vi "PFI-28000-Overload_Create.vi"(0 "String":string, 11 "error in (no error)":errorcluster) -> (4 "PFI-28000-Overload out":refnum<class "PFI-28000-Overload.lvclass">, 15 "error out":errorcluster)   [LabVIEW 2017, in "PFI-28000-Overload.lvclass"]
uses:
  PFI-28000-Overload.lvclass
  PFI-28000-Overload-Type.ctl
  PFI-28000-Overload.lvclass/PFI-28000-Overload.ctl
  <vilib>/regexp/Match Regular Expression.xnode
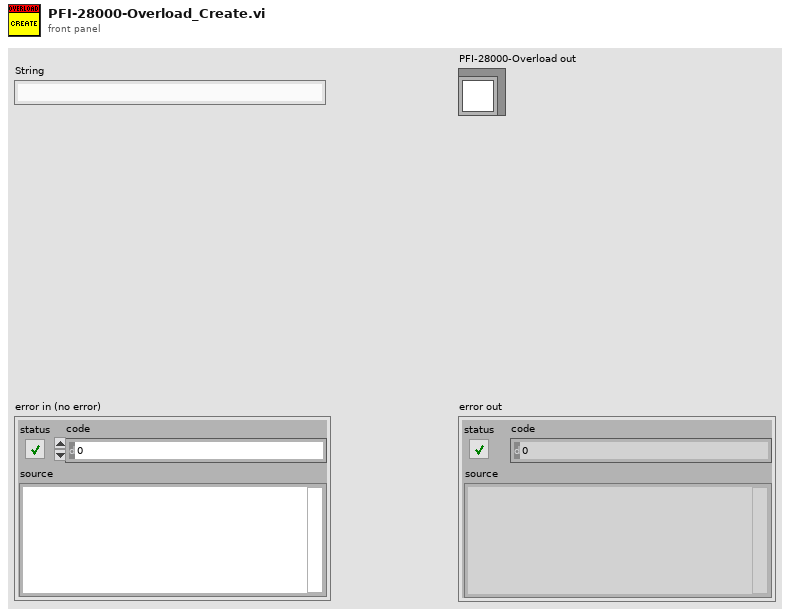
[diagram p1: front panel]
types:
  T1 = typedef "PFI-28000-Overload.lvclass/PFI-28000-Overload-Type.ctl" = enum8{"None", "Filter Input", "Input", "Output", "Open", "Short", "Alarm"}
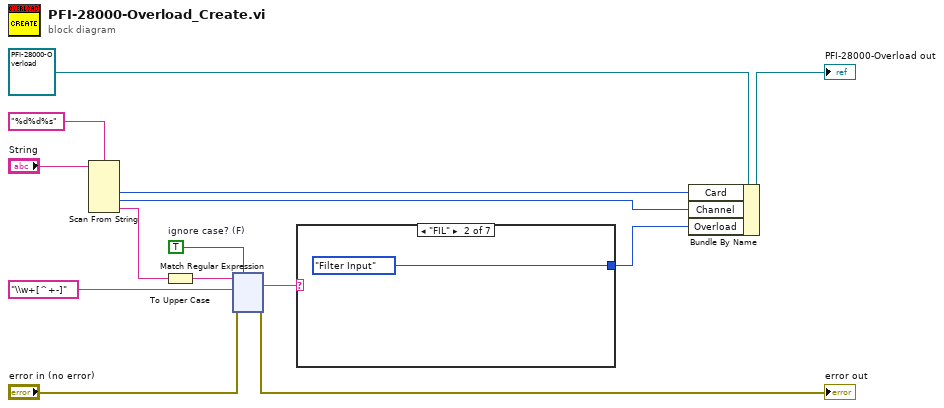
[diagram p0: block diagram]
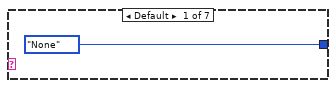
[diagram p2: hidden frame]
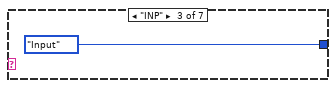
[diagram p3: hidden frame]
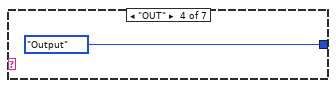
[diagram p4: hidden frame]
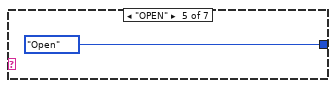
[diagram p5: hidden frame]
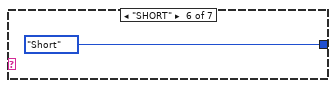
[diagram p6: hidden frame]
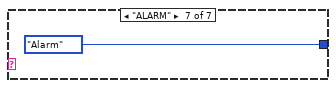
[diagram p7: hidden frame]
diagram:
  w1 = TRUE  # ignore case? (F)
  n1 = Scan From String(format string="%d%d%s" ("empty string"), input string="String") -> (output 1=w11:i32, output 2=w10:i32, output 3=w6:string)  [unwired: 5 in, 3 out]
  n2 = To Upper Case(1:w6) -> (0:w2:string)
  n3 = xnode "Match Regular Expression"("input string"=w2, "regular expression"="\\w+[^+-]" ("empty string"), "error in"="error in (no error)", "ignore case? (F)"=w1) -> ("whole match"=w5:string, "error out"=→"error out":errorcluster)  [unwired: 2 in, 3 out]
  n4 = case shown="\"FIL\"" w5 {
    tunnel: [PFI-28000-Overload-Type."None" ("Overload") PFI-28000-Overload-Type."Filter Input" ("Overload") PFI-28000-Overload-Type."Input" ("Overload") PFI-28000-Overload-Type."Output" ("Overload") PFI-28000-Overload-Type."Open" ("Overload") PFI-28000-Overload-Type."Short" ("Overload") PFI-28000-Overload-Type."Alarm" ("Overload")] -> w8
    frame Default {
    }
    frame "FIL" {
    }
    frame "INP" {
    }
    frame "OUT" {
    }
    frame "OPEN" {
    }
    frame "SHORT" {
    }
    frame "ALARM" {
    }
  }
  n5 = Bundle By Name(cluster=refnum<class "PFI-28000-Overload.lvclass"> refnum ("PFI-28000-Overload in"), "Card"=w11, "Channel"=w10, "Overload"=w8) -> (→"PFI-28000-Overload out":refnum<class "PFI-28000-Overload.lvclass">)
